vi "Line Minimum Derivative.vi"(6 "Parsed Formula":cluster{"table":i32[][], "result":dbl[]}, 7 "Variables":i32[](array[numeric])=[0, 0], 9 "tol":dbl=1e-06 format="%.2e", 10 "p":dbl[](array[numeric]) format="%.2f", 11 "xit":dbl[](array[numeric]) format="%.2f") -> (0 "error":i32, 1 "f(p)":dbl format="%.2f", 2 "pnew":dbl[](array[numeric]) format="%.2f", 3 "xitnew":dbl[](array[numeric]) format="%.2f")   [LabVIEW 2020, in "NI_Gmath.lvlib"]
uses:
  <vilib>/gmath/NI_Gmath.lvlib
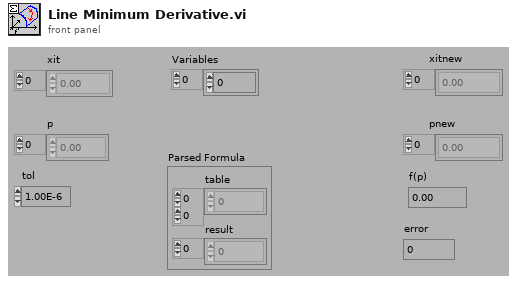
[diagram p1: front panel]
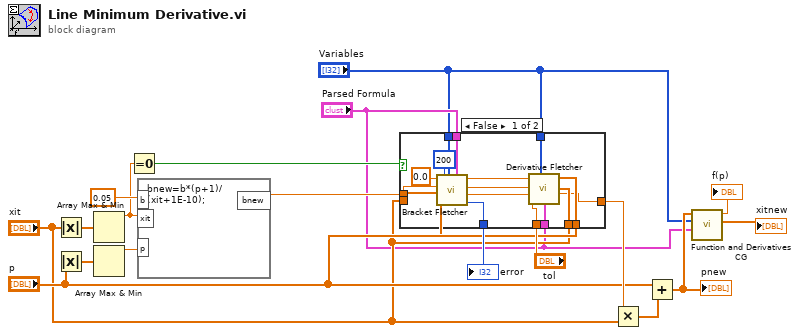
[diagram p0: block diagram]
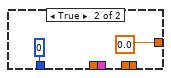
[diagram p2: hidden frame]
diagram:
  n1 = Absolute Value(x="xit") -> (abs(x)=w9:dbl[])
  n2 = Absolute Value(x="p") -> (abs(x)=w8:dbl[])
  n3 = Array Max & Min(array=w9) -> (max value=w5:dbl)  [unwired: 3 out]
  n4 = Array Max & Min(array=w8) -> (max value=w6:dbl)  [unwired: 3 out]
  n5 = Equal To 0?(x=w5) -> (x = 0?=w4:bool)
  n6 = formula code="bnew=b*(p+1)/(xit+1E-10);"("b"=0.05, "xit"=w5, "p"=w6) -> ("bnew"=w11:dbl)
  n7 = case shown="False" w4 {
    tunnel: "p" -> [w32 _]
    tunnel: "xit" -> [w31 _]
    tunnel: w11 -> [w30 _]
    tunnel: [w29 0.0] -> w12
    tunnel: "tol" -> [w28 _]
    tunnel: [w24 0] -> w18
    tunnel: "xit" -> [w23 _]
    tunnel: "Variables" -> [w22 _]
    tunnel: "Parsed Formula" -> [w21 _]
    tunnel: "Variables" -> [w20 _]
    tunnel: "Parsed Formula" -> [w19 _]
    frame False {
      n8 = call <vilib>:"Bracket Fletcher.vi"("Parsed Formula"=w21, "loops"=u32 200, "Variables"=w22, "p"=w32, "xit"=w23, "b (start)"=w30, "a (start)"=0.0) -> ("error"=w24:i32, "c (bracket)"=w27:dbl, "b (bracket)"=w26:dbl, "a (bracket)"=w25:dbl)  [unwired: 1 in]
      n9 = call <vilib>:"Derivative Fletcher.vi"("xi"=w31, "p"=w32, "Parsed Formula"=w19, "Variables"=w20, "ftol"=w28, "c (start)"=w27, "b (start)"=w26, "a (start)"=w25) -> ("x"=w29:dbl)  [unwired: 2 in, 1 out]
    }
    frame True {
    }
  }
  "error" <- w18
  n10 = Multiply(x=w12, y="xit") -> (x*y=w15:dbl[])
  n11 = Add(x="p", y=w15) -> (x+y=w17:dbl[])
  "pnew" <- w17
  n12 = call <vilib>:"Function and Derivatives CG.vi"("Parsed Formula"="Parsed Formula", "Variables"="Variables", "X"=w17) -> ("df/dX"=→"xitnew":dbl[], "f(X)"=→"f(p)":dbl)  [unwired: 7 in]
